vi "WT300 Get Data.vi"(8 "error in (no error)":errorcluster, 11 "VISA resource name":refnum<visa-resource-name>) -> (0 "error out":errorcluster, 1 "Power":sgl caption="Measure Value" format="%.3f", 2 "VISA resource name out":refnum<visa-resource-name>, 3 "Power Data":T1={"Current (A):Element 1"=236.2, "Current (A):Element 2"=17.749, "Power (W):Sigma"=4192.0, "Watt Hours (Wh):Sigma"=0.0, "Voltage (V):Element 2"=236.2, "Voltage (V):Element 1"=236.2, "Current Crest Factor:Element 1"=0.0, "Current Crest Factor:Element 2"=0.0, "Voltage Harmonic (%):Element 1"=0.0, "Voltage Harmonic (%):Element 2"=0.0, "Voltage Crest Factor:Element 1"=0.0, "Voltage Crest Factor:Element 2"=0.0, "Time:Element 1"=0.0, "Frequency (Hz):Element 1"=0.0, "Apparent Power (VA):Element 1"=0.0, "Apparent Power (VA):Element 2"=0.0, "Power Factor:Element 1"=0.0, "Power Factor:Element 2"=0.0, "Max Watt Hours"=0.0, "Voltage (V):Element 2 Avg"=0.0, "Voltage (V):Element 1 Avg"=0.0} {"Voltage (V):Element 1 Avg" format="%.3g"; "Voltage (V):Element 2 Avg" format="%.3g"; "Max Watt Hours" format="%.3g"; "Power Factor:Element 2" format="%.3g"; "Power Factor:Element 1" format="%.3g"; "Apparent Power (VA):Element 2" format="%.3g"; "Apparent Power (VA):Element 1" format="%.3g"; "Frequency (Hz):Element 1" format="%.3g"; "Time:Element 1" format="%.3g"; "Voltage Crest Factor:Element 2" format="%.3g"; "Voltage Crest Factor:Element 1" format="%.3g"; "Voltage Harmonic (%):Element 2" format="%.3g"; "Voltage Harmonic (%):Element 1" format="%.3g"; "Current Crest Factor:Element 2" format="%.3g"; "Current Crest Factor:Element 1" format="%.3g"; "Voltage (V):Element 1" format="%.3g"; "Voltage (V):Element 2" format="%.3g"; "Watt Hours (Wh):Sigma" format="%.3f"; "Power (W):Sigma" format="%.3g"; "Current (A):Element 2" format="%.3g"; "Current (A):Element 1" format="%.3g"}, 5 "Yokogawa Data":string[][](array[string]), 7 "Yokogawa DBL Array":dbl[](array[numeric]))   [LabVIEW 2019]
uses:
  Trunk/Utility/Type Definitions/UTILITY Power Data.ctl
panel:
  in  "Dryer PowerData":T1={"Current (A):Element 1"=236.2, "Current (A):Element 2"=17.749, "Power (W):Sigma"=4192.0, "Watt Hours (Wh):Sigma"=0.0, "Voltage (V):Element 2"=236.2, "Voltage (V):Element 1"=236.2, "Current Crest Factor:Element 1"=0.0, "Current Crest Factor:Element 2"=0.0, "Voltage Harmonic (%):Element 1"=0.0, "Voltage Harmonic (%):Element 2"=0.0, "Voltage Crest Factor:Element 1"=0.0, "Voltage Crest Factor:Element 2"=0.0, "Time:Element 1"=0.0, "Frequency (Hz):Element 1"=0.0, "Apparent Power (VA):Element 1"=0.0, "Apparent Power (VA):Element 2"=0.0, "Power Factor:Element 1"=0.0, "Power Factor:Element 2"=0.0, "Max Watt Hours"=0.0, "Voltage (V):Element 2 Avg"=0.0, "Voltage (V):Element 1 Avg"=0.0} {"Voltage (V):Element 1 Avg" format="%.3g"; "Voltage (V):Element 2 Avg" format="%.3g"; "Max Watt Hours" format="%.3g"; "Power Factor:Element 2" format="%.3g"; "Power Factor:Element 1" format="%.3g"; "Apparent Power (VA):Element 2" format="%.3g"; "Apparent Power (VA):Element 1" format="%.3g"; "Frequency (Hz):Element 1" format="%.3g"; "Time:Element 1" format="%.3g"; "Voltage Crest Factor:Element 2" format="%.3g"; "Voltage Crest Factor:Element 1" format="%.3g"; "Voltage Harmonic (%):Element 2" format="%.3g"; "Voltage Harmonic (%):Element 1" format="%.3g"; "Current Crest Factor:Element 2" format="%.3g"; "Current Crest Factor:Element 1" format="%.3g"; "Voltage (V):Element 1" format="%.3g"; "Voltage (V):Element 2" format="%.3g"; "Watt Hours (Wh):Sigma" format="%.3f"; "Power (W):Sigma" format="%.3g"; "Current (A):Element 2" format="%.3g"; "Current (A):Element 1" format="%.3g"}
  # "Output Data from WT210"
  # "Wh"
  # "V"
  # "A"
  # "V Hz"
  # "W"
  # "PF"
  # "VA"
  # "V CF"
  # "A CF"
  # "WT210 can only take one harmonic reading"
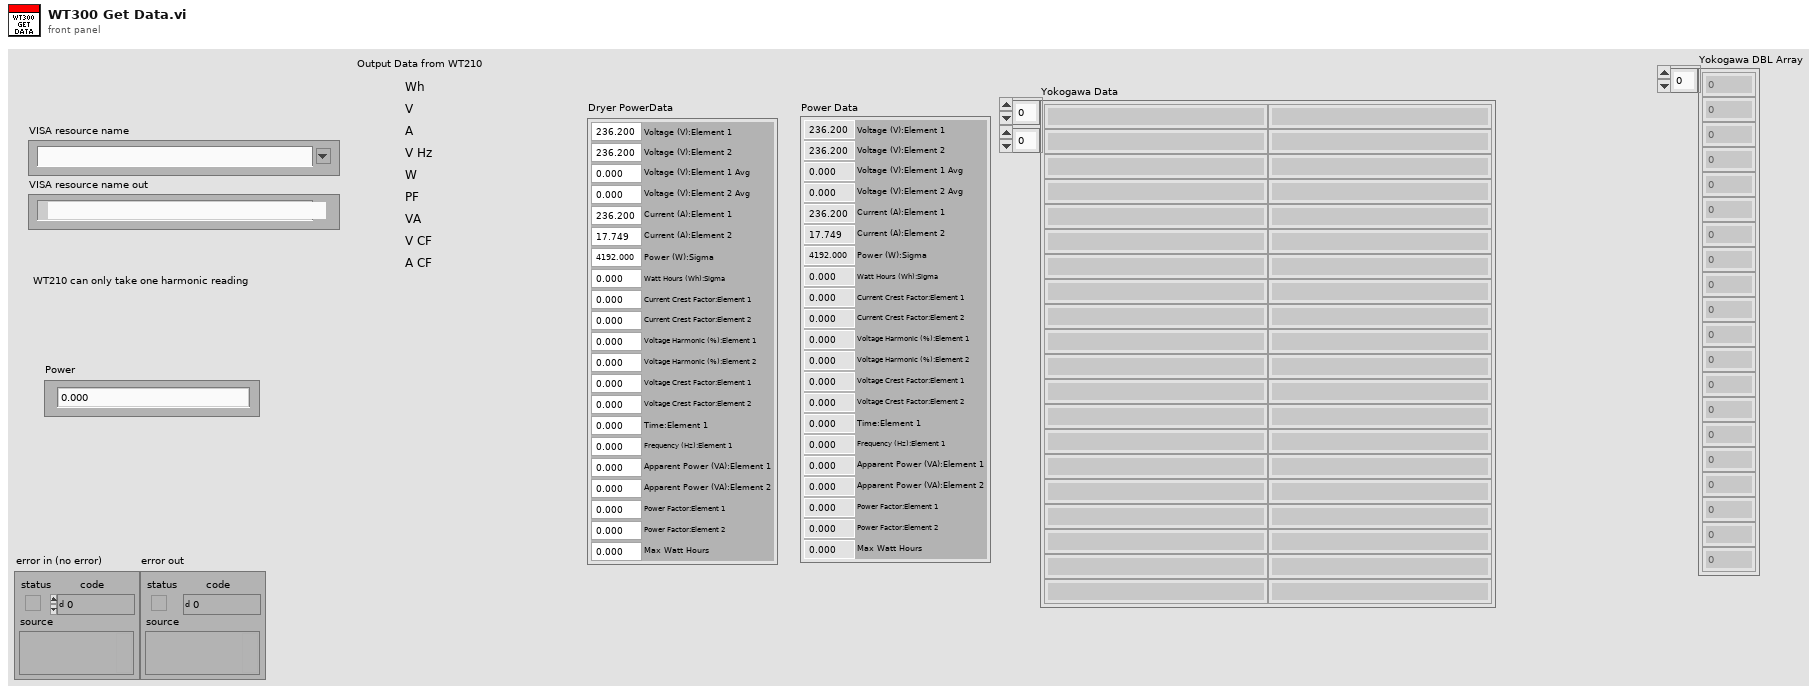
[diagram p1: front panel]
types:
  T1 = typedef "UTILITY Power Data.ctl" = cluster{"Current (A):Element 1":dbl, "Current (A):Element 2":dbl, "Power (W):Sigma":dbl, "Watt Hours (Wh):Sigma":dbl, "Voltage (V):Element 2":dbl, "Voltage (V):Element 1":dbl, "Current Crest Factor:Element 1":dbl, "Current Crest Factor:Element 2":dbl, "Voltage Harmonic (%):Element 1":dbl, "Voltage Harmonic (%):Element 2":dbl, "Voltage Crest Factor:Element 1":dbl, "Voltage Crest Factor:Element 2":dbl, "Time:Element 1":dbl, "Frequency (Hz):Element 1":dbl, "Apparent Power (VA):Element 1":dbl, "Apparent Power (VA):Element 2":dbl, "Power Factor:Element 1":dbl, "Power Factor:Element 2":dbl, "Max Watt Hours":dbl, "Voltage (V):Element 2 Avg":dbl, "Voltage (V):Element 1 Avg":dbl}
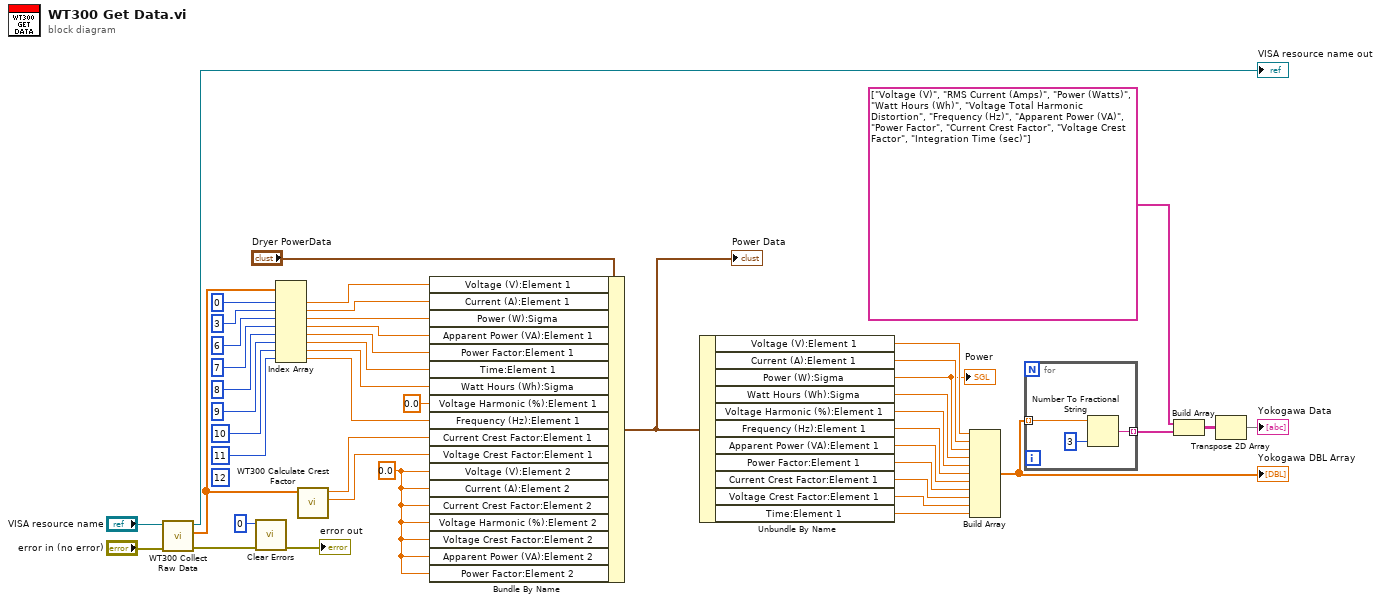
[diagram p0: block diagram]
diagram:
  (unwired) 12 ("index")
  w13 = 0.0 ("Urms:Element 2")
  n1 = call "WT300 Collect Raw Data.vi"("error in (no error)"="error in (no error)", "VISA Refnum in"="VISA resource name") -> ("error out"=w5:errorcluster, "Data"=w15:dbl[], "VISA resource name out"=→"VISA resource name out":refnum<visa-resource-name>)  [unwired: 6 in, 1 out]
  n2 = call <vilib>:"Clear Errors.vi"("error in (no error)"=w5, "specific error code to clear (0: all)"=0) -> ("error out"=→"error out":errorcluster)  [unwired: 4 in, 1 out]
  n3 = Index Array(array=w15, index #1=0 ("index"), index #2=3 ("index"), index #3=6 ("index"), index #4=7 ("index"), index #5=8 ("index"), index #6=9 ("index"), index #7=10 ("index"), index #8=11 ("index")) -> (element #1=w26:dbl, element #2=w24:dbl, element #3=w22:dbl, element #4=w12:dbl, element #5=w11:dbl, element #6=w10:dbl, element #7=w17:dbl, element #8=w2:dbl)
  n4 = call "WT300 Calculate Crest Factor.vi"("All Data"=w15) -> ("Voltage Crest Factor"=w8:dbl, "Current Crest Factor"=w9:dbl)  [unwired: 9 in]
  n5 = Bundle By Name(cluster="Dryer PowerData", "Voltage (V):Element 1"=w26, "Current (A):Element 1"=w24, "Power (W):Sigma"=w22, "Apparent Power (VA):Element 1"=w12, "Power Factor:Element 1"=w11, "Time:Element 1"=w10, "Watt Hours (Wh):Sigma"=w17, "Voltage Harmonic (%):Element 1"=0.0, "Frequency (Hz):Element 1"=w2, "Current Crest Factor:Element 1"=w9, "Voltage Crest Factor:Element 1"=w8, "Voltage (V):Element 2"=w13, "Current (A):Element 2"=w13, "Current Crest Factor:Element 2"=w13, "Voltage Harmonic (%):Element 2"=w13, "Voltage Crest Factor:Element 2"=w13, "Apparent Power (VA):Element 2"=w13, "Power Factor:Element 2"=w13) -> (w43:T1)
  "Power Data" <- w43
  n6 = Unbundle By Name(w43) -> ("Voltage (V):Element 1"=w42:dbl, "Current (A):Element 1"=w41:dbl, "Power (W):Sigma"=w27:dbl, "Watt Hours (Wh):Sigma"=w40:dbl, "Voltage Harmonic (%):Element 1"=w39:dbl, "Frequency (Hz):Element 1"=w38:dbl, "Apparent Power (VA):Element 1"=w37:dbl, "Power Factor:Element 1"=w36:dbl, "Current Crest Factor:Element 1"=w35:dbl, "Voltage Crest Factor:Element 1"=w34:dbl, "Time:Element 1"=w29:dbl)
  "Power" <- w27
  n7 = Build Array(w42, w41, w27, w40, w39, w38, w37, w36, w35, w34, w29) -> (w31:dbl[])
  "Yokogawa DBL Array" <- w31
  n8 = for {
    tunnel: w31 -> [w47] mode=indexing
    tunnel: [w46] -> w7 mode=indexing
    n9 = Number To Fractional String(number=w47, precision (6)=i16 3) -> (F-format string=w46:string)  [unwired: 2 in]
  }
  n10 = Build Array(string[] ["Voltage (V)", "RMS Current (Amps)", "Power (Watts)", "Watt Hours (Wh)", "Voltage Total Harmonic Distortion", "Frequency (Hz)", "Apparent Power (VA)", "Power Factor", "Current Crest Factor", "Voltage Crest Factor", "Integration Time (sec)"], w7) -> (w6:string[][])
  n11 = Transpose 2D Array(2D array=w6) -> (transposed array=→"Yokogawa Data":string[][])
